vi "Create Listener.vi"(8 "Error In":errorcluster, 11 "Port Number":i32=4001) -> (0 "Error Out":errorcluster, 3 "Listener":refnum<k24>)   [LabVIEW 2014, in "SSL Lib.lvlib"]
doc: "VI Function: This VI starts a TCP listener to the input port number.\n\nVI Version: 1.0\n\nVI Author: Runjhun Agarwal"
uses:
  <userlib>/SSL Library/SSL Lib.lvlib
  <userlib>/SSL Library/Controls/Ref.ctl
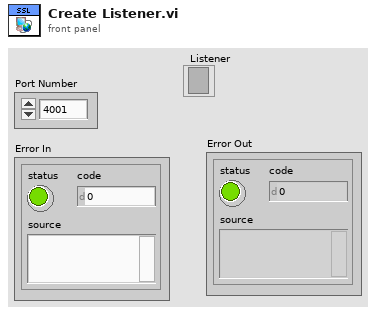
[diagram p1: front panel]
types:
  T1 = typedef "Ref.ctl" = enum16{"Update Ref", "Read Ref", "Close Ref"}
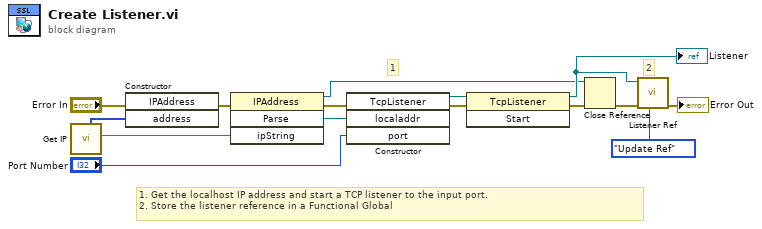
[diagram p0: block diagram]
diagram:
  # "1"
  # "2"
  # "1. Get the localhost IP address and start a TCP listener to the input port.\n2. Store the listener reference in a Functional Global"
  n1 = call <userlib>:"Get IP.vi"() -> ("IP Address"=w9:string, "IP Address(Bytes)"=w10:u8[])  [unwired: 10 in]
  n2 = constructor class="IPAddress"(error in="Error In", "address"=w10) -> (error out=w14:errorcluster)  [unwired: 2 in, 3 out]
  n3 = invoke class="IPAddress" method="Parse"(error in=w14, "ipString"=w9) -> (reference out=w5:refnum<k24>, error out=w1:errorcluster, "Parse"=w4:refnum<k24>)  [unwired: 2 in, 1 out]
  n4 = constructor class="TcpListener"(error in=w1, "localaddr"=w4, "port"="Port Number") -> (reference out=w11:refnum<k24>, error out=w12:errorcluster)  [unwired: 2 in, 3 out]
  n5 = invoke class="TcpListener" method="Start"(reference=w11, error in=w12) -> (reference out=w8:refnum<k24>, error out=w3:errorcluster)  [unwired: 1 in, 1 out]
  "Listener" <- w8
  n6 = Close Reference(reference=w5, error in (no error)=w3) -> (error out=w2:errorcluster)
  n7 = call <userlib>:"Listener Ref.vi"("Action"=Ref."Update Ref", "Error In"=w2, "Listener Ref"=w8) -> ("Error Out"=→"Error Out":errorcluster)  [unwired: 7 in, 1 out]
